vi "Формулы ПП.vi"(1 "PerB":dbl, 2 "PerA":dbl, 3 "mode":i32) -> (0 "Exid":dbl)   [LabVIEW 2018]
uses:
  qwerty.dll
panel:
  # "5 Формул\n1 - объем V=(pi*D^2 )/4*L\n2,3 -P=m/V \n4 - Пористость=(Vp/V)*100\n5 - Vc = V-Vp"
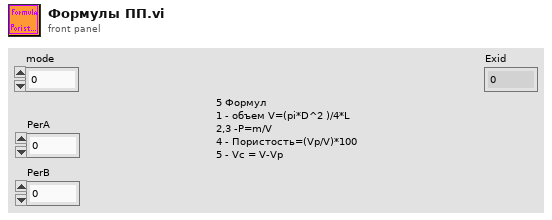
[diagram p1: front panel]
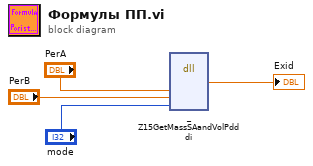
[diagram p0: block diagram]
diagram:
  n1 = dll-call lib="C:/Users/serg1/Documents/LabVIEW Data/Project)/qwerty.dll" fn="_Z15GetMassSAandVolPdddi"("PerA"="PerA", "PerB"="PerB", "mode"="mode") -> ("Exid"=→"Exid":dbl)  [unwired: 8 in, 2 out]
